vi "Plant1_model.vi"(10 "Input = u(t)":dbl) -> (2 "State = x(t)":dbl[](array[numeric]))   [LabVIEW 2016]
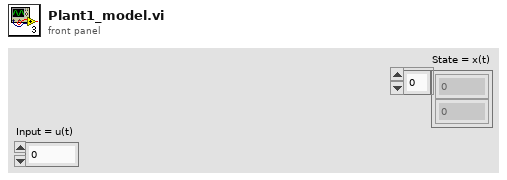
[diagram p1: front panel]
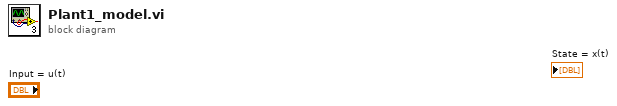
[diagram p0: block diagram]
diagram:
